vi "Demo v8_QL.vi"() -> ()   [LabVIEW 2013]
panel:
  out "Boolean 4":bool
  out "Boolean 3":bool
  out "Boolean 2":bool
  out "Boolean":bool
  in  "Q 4":bool
  out "Last 5 scores":i32
  in  "Q 3":bool
  in  "Q 2":bool
  in  "Q 1":bool
  out "Best Score":i32
  out "Jump":bool
  in  "AI":bool=TRUE
  in  "Jump":bool
  out "Fail":bool
  in  "Speed":u32(slide)=25 scale=15.0..40.0
  in  "Re-study":bool
  in  "stop":bool
  out "Score":i32
  out "Picture":i32[][](graph)
  # "Flappy Bird\nChallenge"
  # "AI \nReinforcement\nLearning"
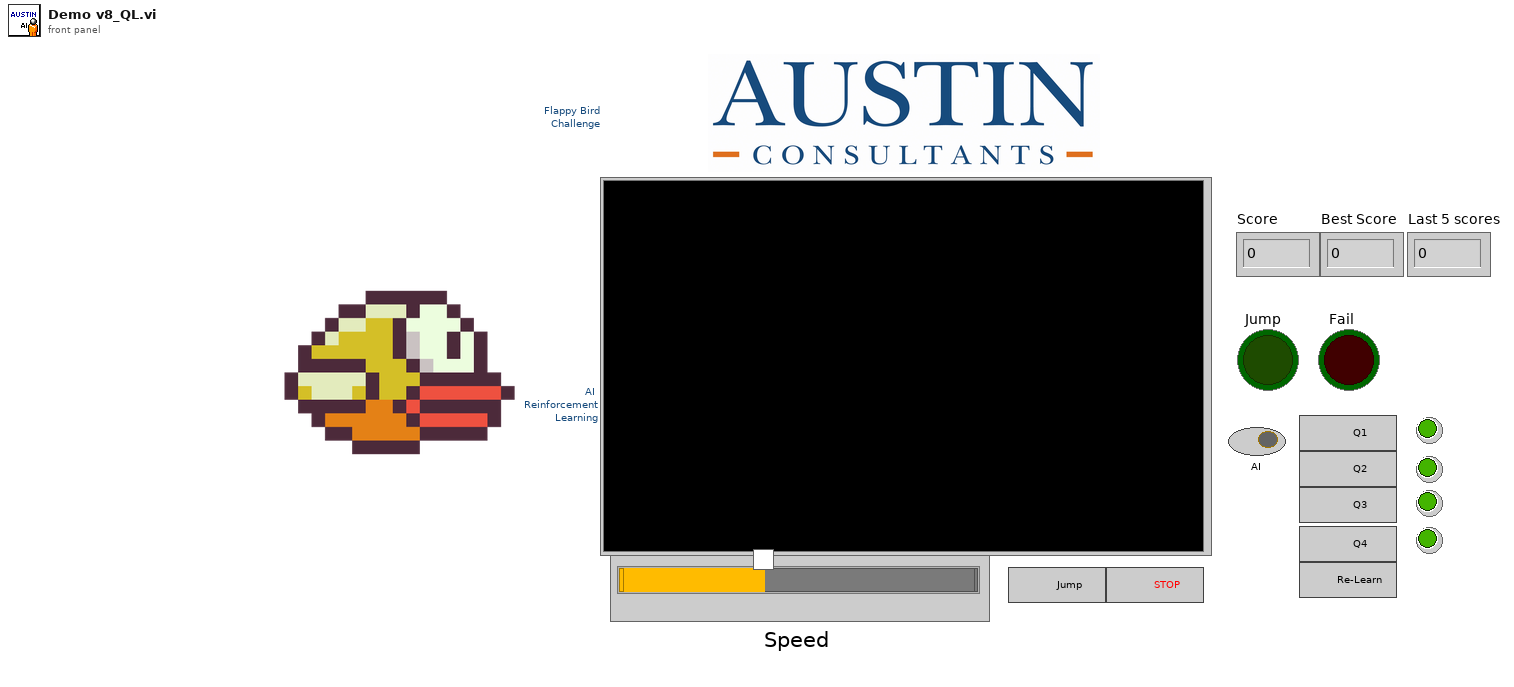
[diagram p1: front panel]
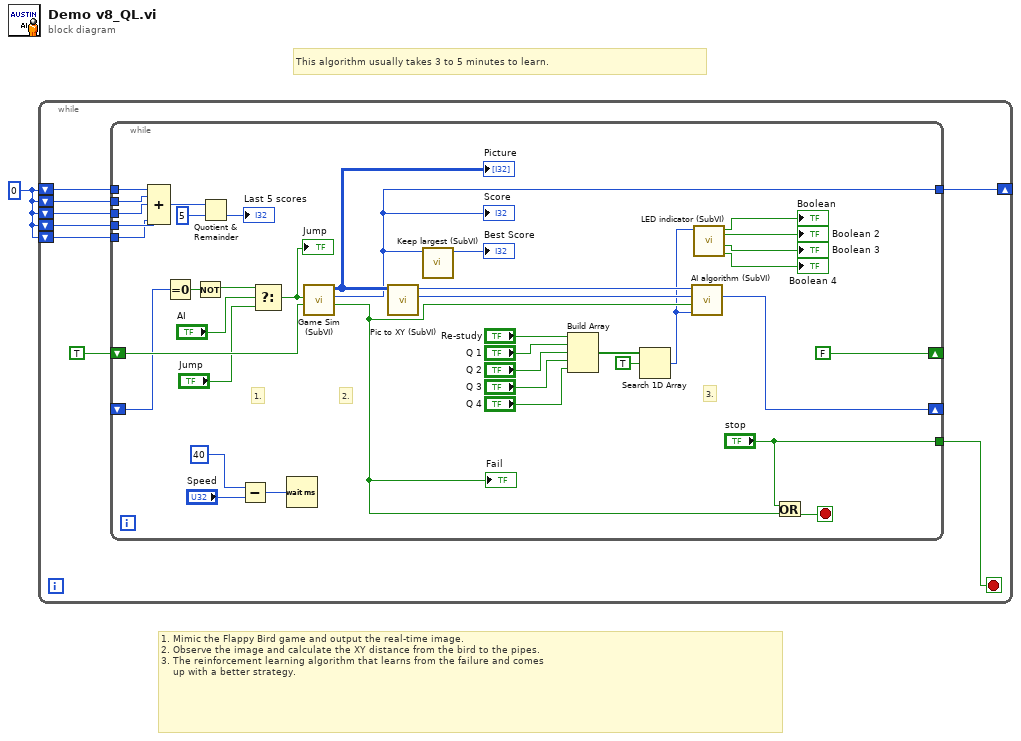
[diagram p0: block diagram]
diagram:
  w1 = 0 ("Score")
  # "1. Mimic the Flappy Bird game and output the real-time image.\n2. Observe the image and calculate the XY distance from the bird to the pipes.\n3. The reinforcement learning algorithm that learns from the failure and comes\n    up with a better strategy."
  # "This algorithm usually takes 3 to 5 minutes to learn."
  n1 = while {
    shift-right: [w7] -> _
    shift-left: w1 -> [w6]
    shift-left: w1 -> [w5]
    shift-left: w1 -> [w4]
    shift-left: w1 -> [w3]
    shift-left: w1 -> [w2]
    stop <- w8 stop-if-true
    n2 = while {
      shift-right: [FALSE ("Reset")] -> _
      shift-left: TRUE ("Reset") -> [w49]
      shift-right: [w41] -> _
      shift-left: _ -> [w45]
      tunnel: ["stop"] -> w8
      tunnel: [w24] -> w7
      tunnel: w6 -> [w23]
      tunnel: w5 -> [w22]
      tunnel: w4 -> [w21]
      tunnel: w3 -> [w20]
      tunnel: w2 -> [w19]
      stop <- w35 stop-if-true
      # "3."
      # "2."
      # "1."
      n3 = Compound Arithmetic op=unknown(w23, w22, w21, w20, w19) -> (w18:i32)
      n4 = Equal To 0?(x=w45) -> (x = 0?=w46:bool)
      n5 = Not(x=w46) -> (.not. x?=w38:bool)
      n6 = Quotient & Remainder(x=w18, y=5) -> (floor(x/y)=→"Last 5 scores":i32)  [unwired: 1 out]
      n7 = Subtract(x=u32 40, y="Speed") -> (x-y=w43:u32)
      n8 = Select(t=w38, s="AI", f="Jump") -> (s? t:f=w36:bool)
      "Jump" <- w36
      n9 = Wait (ms)(milliseconds to wait=w43) -> ()  [unwired: 1 out]
      n10 = call "Game Sim (SubVI).vi"("Reset"=w49, "Jump"=w36) -> ("Fail"=w40:bool, "Score"=w24:i32, "Picture"=w47:i32[][])  [unwired: 7 in]
      "Picture" <- w47
      "Score" <- w24
      "Fail" <- w40
      n11 = call "Pic to XY (SubVI).vi"("Picture"=w47) -> ("Y distance"=w32:i32, "X distance"=w33:i32)  [unwired: 9 in]
      n12 = call "Keep largest (SubVI).vi"("Input"=w24) -> ("Biggest"=→"Best Score":i32)  [unwired: 10 in]
      n13 = Build Array("Re-study", "Q 1", "Q 2", "Q 3", "Q 4") -> (w30:bool[])
      n14 = Search 1D Array(1D array=w30, element=TRUE) -> (index of element=w14:i32)  [unwired: 1 in]
      n15 = call "AI algorithm (SubVI).vi"("Q option"=w14, "Jump?"=w40, "y"=w32, "x"=w33) -> ("Next Action"=w41:i32)  [unwired: 6 in, 1 out]
      n16 = call "LED indicator (SubVI).vi"("index of element"=w14) -> ("Boolean 4"=→"Boolean 4":bool, "Boolean 3"=→"Boolean 3":bool, "Boolean 2"=→"Boolean 2":bool, "Boolean"=→"Boolean":bool)  [unwired: 7 in]
      n17 = Or(x="stop", y=w40) -> (x .or. y?=w35:bool)
    }
  }
